vi "test_Monitor - FPGA to Host.vi"(8 "error in (no error)":errorcluster, 11 "IO Data_Rd":u32[](array[numeric]) format="%.0x") -> (0 "error out":errorcluster, 3 "Monitor IO Data":u32[](array[numeric]) format="%.0x")   [LabVIEW 2016]
uses:
  Host/Typedefs/Monitor Data Operation.ctl
  Host/Typedefs/LV2G Operation.ctl
  Host/Typedefs/IO Buffer Operation.ctl
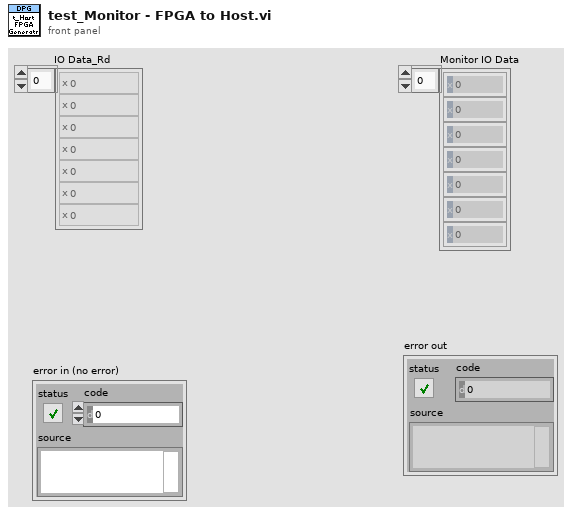
[diagram p1: front panel]
types:
  T1 = typedef "LV2G Operation.ctl" = enum16{"Initialize", "Set", "Get", "Close"}
  T2 = typedef "Monitor Data Operation.ctl" = enum16{"Obtain", "Enqueue", "Read Elements", "Flush", "Release", "Read Last Element"}
  T3 = typedef "IO Buffer Operation.ctl" = enum16{"Initialize", "Write IO Data_Rd", "Read IO Data_Rd", "Write IO Data_Wr", "Read IO Data_Wr", "Write  IO Data_Dir", "Read  IO Data_Dir", "Write Host to Target FIFO", "Read Host to Target FIFO", "Write Target to Host FIFO", "Read Target to Host FIFO", "Write Monitor Enable?", "Read Monitor Enable?", "Close"}
  T4 = typedef "Monitor Data Element.ctl" = cluster{"Pin Data":u32, "Transition ":u32}
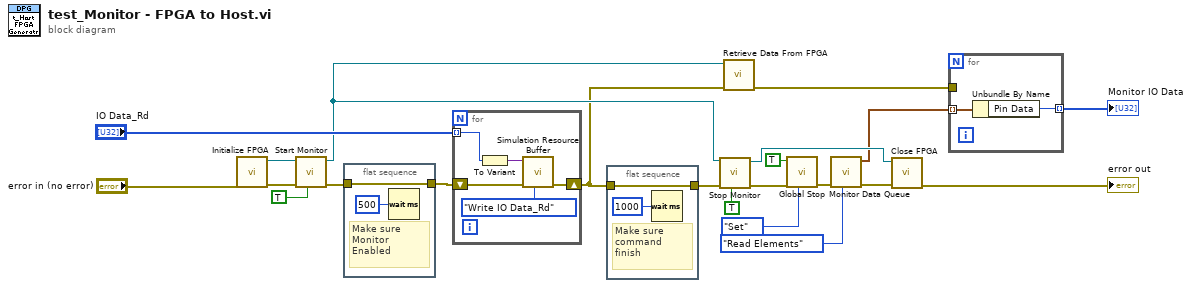
[diagram p0: block diagram]
diagram:
  n1 = call "Initialize FPGA.vi"("error in (no error)"="error in (no error)") -> ("error out"=w22:errorcluster, "FPGA VI Reference"=w21:refnum<k20>)  [unwired: 9 in]
  n2 = call "Start Monitor.vi"("Write to FPGA(T)"=TRUE, "error in (no error)"=w22, "FPGA VI Reference In"=w21) -> ("error out"=w6:errorcluster, "FPGA VI Reference out"=w16:refnum<k20>)  [unwired: 7 in]
  n3 = flat-sequence {
    tunnel: w6 -> [w23]
    tunnel: [w23] -> w5
    frame #0 {
      # "Make sure \nMonitor Enabled"
      n4 = Wait (ms)(milliseconds to wait=u32 500) -> ()  [unwired: 1 out]
    }
  }
  n5 = for {
    tunnel: "IO Data_Rd" -> [w28] mode=indexing
    shift-right: [w25] -> w4
    shift-left: w5 -> [w29]
    n6 = To Variant(anything=w28) -> (Variant=w27:variant)
    n7 = call "Simulation Resource Buffer.vi"("IO Buffer Operation"=IO_Buffer_Operation."Write IO Data_Rd", "error in (no error)"=w29, "Data in"=w27) -> ("error out"=w25:errorcluster)  [unwired: 6 in, 2 out]
  }
  n8 = flat-sequence {
    tunnel: w4 -> [w30]
    tunnel: [w30] -> w3
    frame #0 {
      # "Make sure \ncommand \nfinish"
      n9 = Wait (ms)(milliseconds to wait=u32 1000) -> ()  [unwired: 1 out]
    }
  }
  n10 = call "Stop Monitor.vi"("Write to FPGA(T)"=TRUE, "error in (no error)"=w3, "FPGA VI Reference In"=w16) -> ("error out"=w8:errorcluster, "FPGA VI Reference Out"=w19:refnum<k20>)  [unwired: 7 in]
  n11 = call "Retrieve Data From FPGA.vi"("error in (no error)"=w4, "FPGA VI Reference In"=w16) -> ("error out"=w9:errorcluster)  [unwired: 9 in]
  n12 = call "Global Stop.vi"("Stop Operation (Get)"=LV2G_Operation."Set", "error in (no error)"=w8, "Stop?"=TRUE) -> ("error out"=w14:errorcluster)  [unwired: 7 in, 1 out]
  n13 = call "Monitor Data Queue.vi"("Queue Function"=Monitor_Data_Operation."Read Elements", "error in (no error)"=w14) -> ("error out"=w7:errorcluster, "Queue Elements"=w11:T4[])  [unwired: 6 in, 2 out]
  n14 = call "Close FPGA.vi"("error in (no error)"=w7, "Refnum in"=w19) -> ("error out"=→"error out":errorcluster)  [unwired: 9 in]
  n15 = for {
    tunnel: w11 -> [w33] mode=indexing
    tunnel: [w32] -> w10 mode=indexing
    tunnel: w9 -> [_]
    n16 = Unbundle By Name(w33) -> ("Pin Data"=w32:u32)
  }
  "Monitor IO Data" <- w10
